vi "Temperature Check.vi"(8 "error in (no error)":errorcluster, 10 "WaitMoniter Input":T4={"Wait Time(S)"=10.0, "Chamber Temp(Deg C)"=10.0, "Chamber Temp Tolerance(%)"=10.0, "RMS Current(A)"=10.0, "RMS Current Tolerance(%)"=10.0, "Temperature Control"=FALSE, "RMS Control"=FALSE, "RMS Current Min(A)"=10.0, "RMS Current Max(A)"=10.0, "Chamber Temp Min(Deg C)"=10.0, "Chamber Temp Max(Deg C)"=10.0, "HVPPS Current Max(A)"=10.0, "HVPPS Control"=FALSE, "HVPPS Current(A)"=10.0} {"HVPPS Current(A)" format="%#_13g"; "HVPPS Current Max(A)" format="%#_13g"; "Chamber Temp Max(Deg C)" format="%#_13g"; "Chamber Temp Min(Deg C)" format="%#_13g"; "RMS Current Max(A)" format="%#_13g"; "RMS Current Min(A)" format="%#_13g"; "RMS Current Tolerance(%)" format="%#_13g"; "RMS Current(A)" format="%#_13g"; "Chamber Temp Tolerance(%)" format="%#_13g"; "Chamber Temp(Deg C)" format="%#_13g"; "Wait Time(S)" format="%#_13g"}, 11 "Data Cluster":T1={"Chamber Address"={"Starting Address"=0, "Data Length"=0}, "Modbus RTU"={"unit ID"=1, "serial type"=enum."RTU", "baud rate"=9600, "parity (even)"=2, "flow control (none)"=0, "VISA resource name"=""}, "Temparature PASS?"=FALSE, "RMS Current PASS?"=FALSE, "Ping PASS?"=FALSE, "WaitMonitor_Class"=refnum, "Status Update"="", "Test Mode"=0, "Sequence Context"=refnum, "Running?"=FALSE, "RMS_FAIL_Count"=0, "Current Temperature"=0.0, "Target Temperature"=0.0, "RMS_Current"=[], "PowerStatus"={"Chamber IP Ping"=FALSE, "RAW_Power_Status"=FALSE, "PDU1_Status_Instrument_Rack"=FALSE, "PDU2_Status_PowerSupply_Rack_1"=FALSE, "PDU3_Status_PowerSupply_Rack_2"=FALSE}, "Monitor_Interval(S)"=0.0, "Current_Monitor_Interval(S)"=0.0, "RMS_Refresh?"=FALSE, "RTD Temperature(Deg C)"=0.0, "AbortTime(S)"=0.0, "HVPPS_Current"=[], "HVPPS Current PASS?"=FALSE} {"Modbus RTU"."parity (even)" items=["None", "Odd", "Even", "Mark", "Space"]; "Modbus RTU"."flow control (none)" items=["None", "XON/XOFF", "RTS/CTS", "XON/XOFF & RTS/CTS", "DTR/DSR", "XON/XOFF & DTR/DSR"]}) -> (0 "error out":errorcluster, 3 "Data Cluster out":T1={"Chamber Address"={"Starting Address"=0, "Data Length"=0}, "Modbus RTU"={"unit ID"=1, "serial type"=enum."RTU", "baud rate"=9600, "parity (even)"=2, "flow control (none)"=0, "VISA resource name"=""}, "Temparature PASS?"=FALSE, "RMS Current PASS?"=FALSE, "Ping PASS?"=FALSE, "WaitMonitor_Class"=refnum, "Status Update"="", "Test Mode"=0, "Sequence Context"=refnum, "Running?"=FALSE, "RMS_FAIL_Count"=0, "Current Temperature"=0.0, "Target Temperature"=0.0, "RMS_Current"=[], "PowerStatus"={"Chamber IP Ping"=FALSE, "RAW_Power_Status"=FALSE, "PDU1_Status_Instrument_Rack"=FALSE, "PDU2_Status_PowerSupply_Rack_1"=FALSE, "PDU3_Status_PowerSupply_Rack_2"=FALSE}, "Monitor_Interval(S)"=0.0, "Current_Monitor_Interval(S)"=0.0, "RMS_Refresh?"=FALSE, "RTD Temperature(Deg C)"=0.0, "AbortTime(S)"=0.0, "HVPPS_Current"=[], "HVPPS Current PASS?"=FALSE} {"Modbus RTU"."parity (even)" items=["None", "Odd", "Even", "Mark", "Space"]; "Modbus RTU"."flow control (none)" items=["None", "XON/XOFF", "RTS/CTS", "XON/XOFF & RTS/CTS", "DTR/DSR", "XON/XOFF & DTR/DSR"]})   [LabVIEW 2023, in "HardwareAbstractionLayer_LVOOP.lvlib" / "Wait Monitor.lvclass"]
uses:
  Wait Monitor.lvclass
  Control/Data Cluster.ctl
  <vilib>/addons/TestStand/_TSLegacy.llb/LabVIEW Test - Sequence Context.ctl
  Teststand Steptypes/PowerMonitor/Control/PowerData.ctl
  Teststand Steptypes/WaitMoniter/Control/Moniter Step Control.ctl
  Teststand Steptypes/GlobalVariable/GlobalVariableData.vi
  Wait Monitor.lvclass/Wait Monitor.ctl
  Teststand Steptypes/LTT_TeststandSteptypes.lvlib
  <userlib>/_OpenG.lib/error/error.llb/openg_error.lvlib
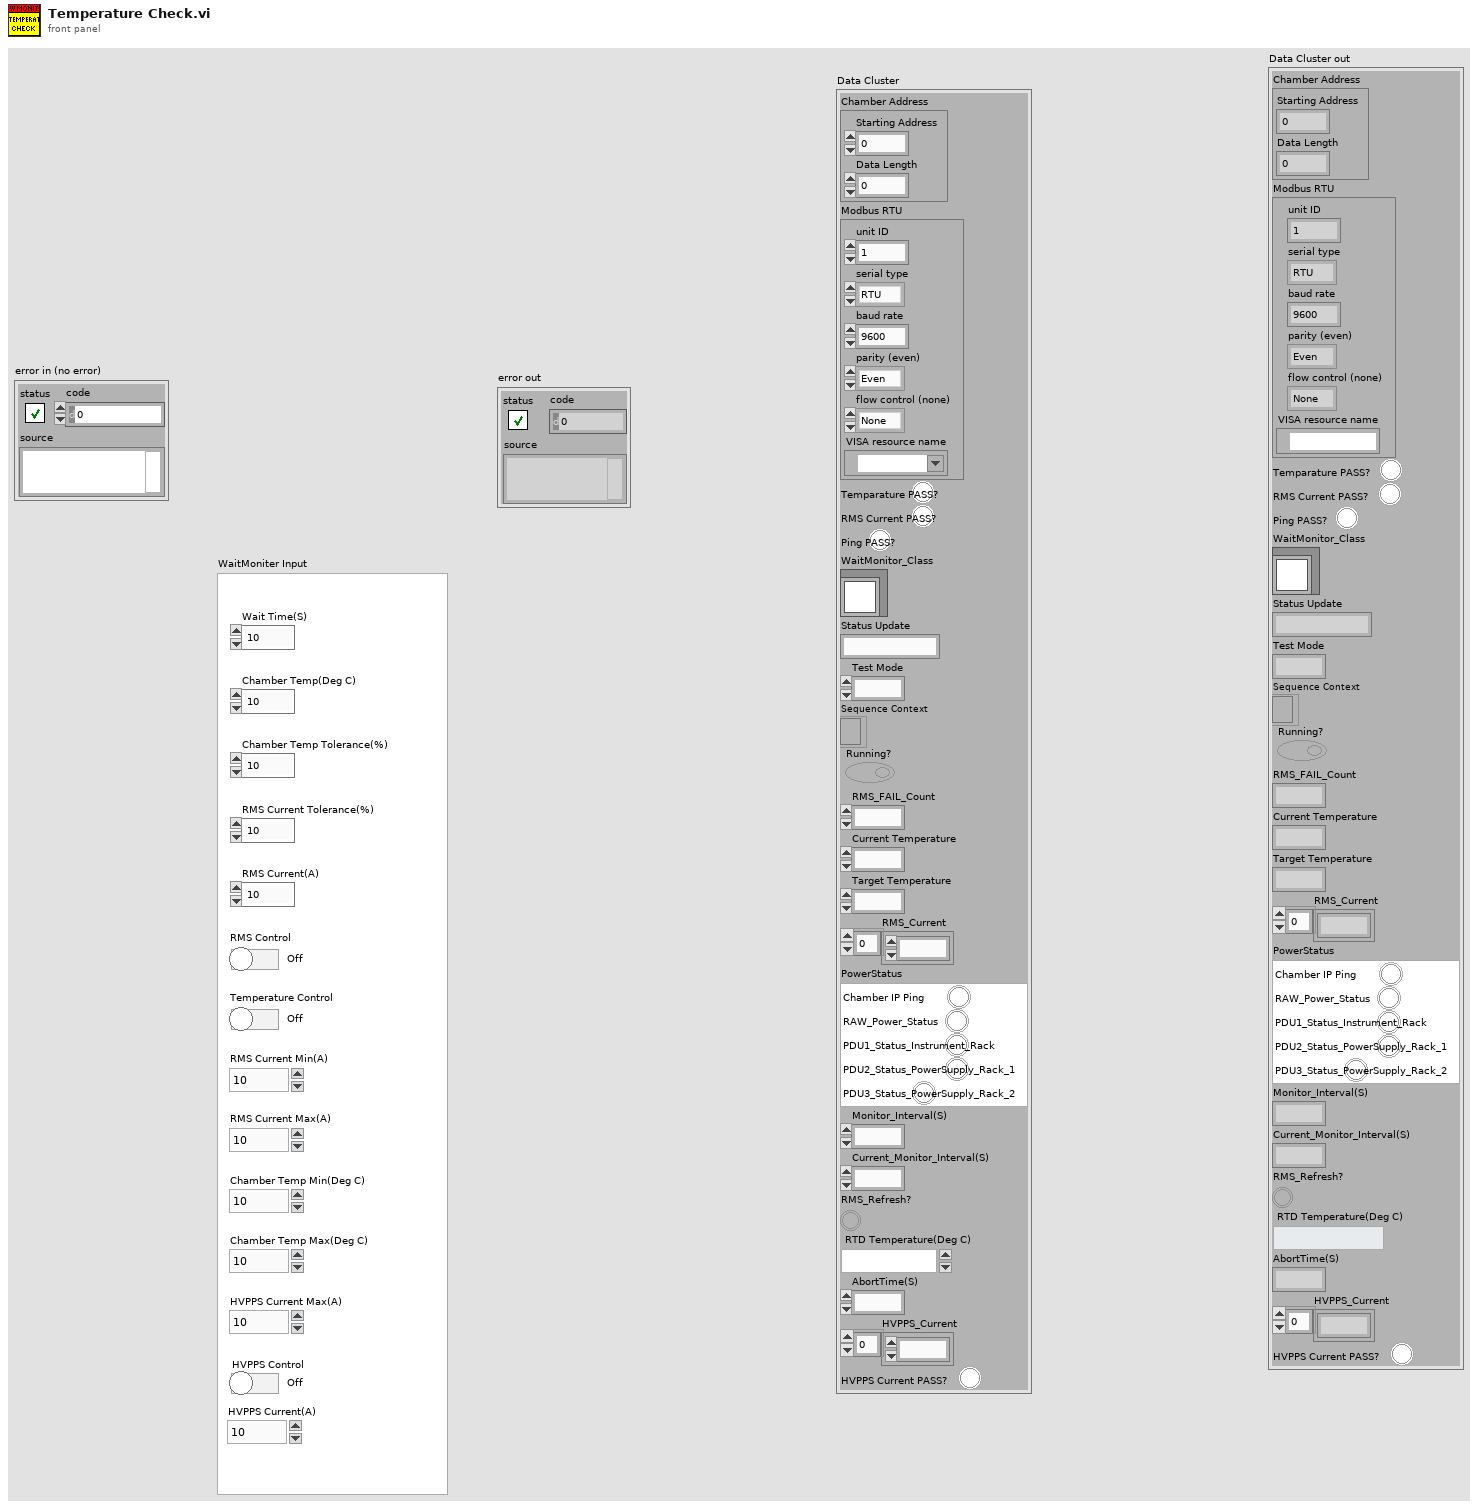
[diagram p1: front panel]
types:
  T1 = typedef "HardwareAbstractionLayer_LVOOP.lvlib/Wait Monitor.lvclass/Data Cluster.ctl" = cluster{"Chamber Address":cluster{"Starting Address":u16, "Data Length":u16}, "Modbus RTU":cluster{"unit ID":u8, "serial type":enum16{"RTU", "ASCII"}, "baud rate":u32, "parity (even)":u16, "flow control (none)":u16, "VISA resource name":refnum<visa-resource-name>}, "Temparature PASS?":bool, "RMS Current PASS?":bool, "Ping PASS?":bool, "WaitMonitor_Class":refnum<class "Wait Monitor.lvclass">, "Status Update":string, "Test Mode":u16, "Sequence Context":T2, "Running?":bool, "RMS_FAIL_Count":u16, "Current Temperature":dbl, "Target Temperature":dbl, "RMS_Current":dbl[], "PowerStatus":T3, "Monitor_Interval(S)":dbl, "Current_Monitor_Interval(S)":dbl, "RMS_Refresh?":bool, "RTD Temperature(Deg C)":dbl, "AbortTime(S)":dbl, "HVPPS_Current":dbl[], "HVPPS Current PASS?":bool}
  T2 = typedef "LabVIEW Test - Sequence Context.ctl" = refnum<k7>
  T3 = typedef "LTT_TeststandSteptypes.lvlib/PowerData.ctl" = cluster{"Chamber IP Ping":bool, "RAW_Power_Status":bool, "PDU1_Status_Instrument_Rack":bool, "PDU2_Status_PowerSupply_Rack_1":bool, "PDU3_Status_PowerSupply_Rack_2":bool}
  T4 = typedef "HardwareAbstractionLayer_LVOOP.lvlib/Wait Monitor.lvclass/Moniter Step Control.ctl" = cluster{"Wait Time(S)":dbl, "Chamber Temp(Deg C)":dbl, "Chamber Temp Tolerance(%)":dbl, "RMS Current(A)":dbl, "RMS Current Tolerance(%)":dbl, "Temperature Control":bool, "RMS Control":bool, "RMS Current Min(A)":dbl, "RMS Current Max(A)":dbl, "Chamber Temp Min(Deg C)":dbl, "Chamber Temp Max(Deg C)":dbl, "HVPPS Current Max(A)":dbl, "HVPPS Control":bool, "HVPPS Current(A)":dbl}
  T5 = cluster{"Chamber Present Temp":dbl, "Chamber Target Temp":dbl, "Chamber RTD Temp":dbl}
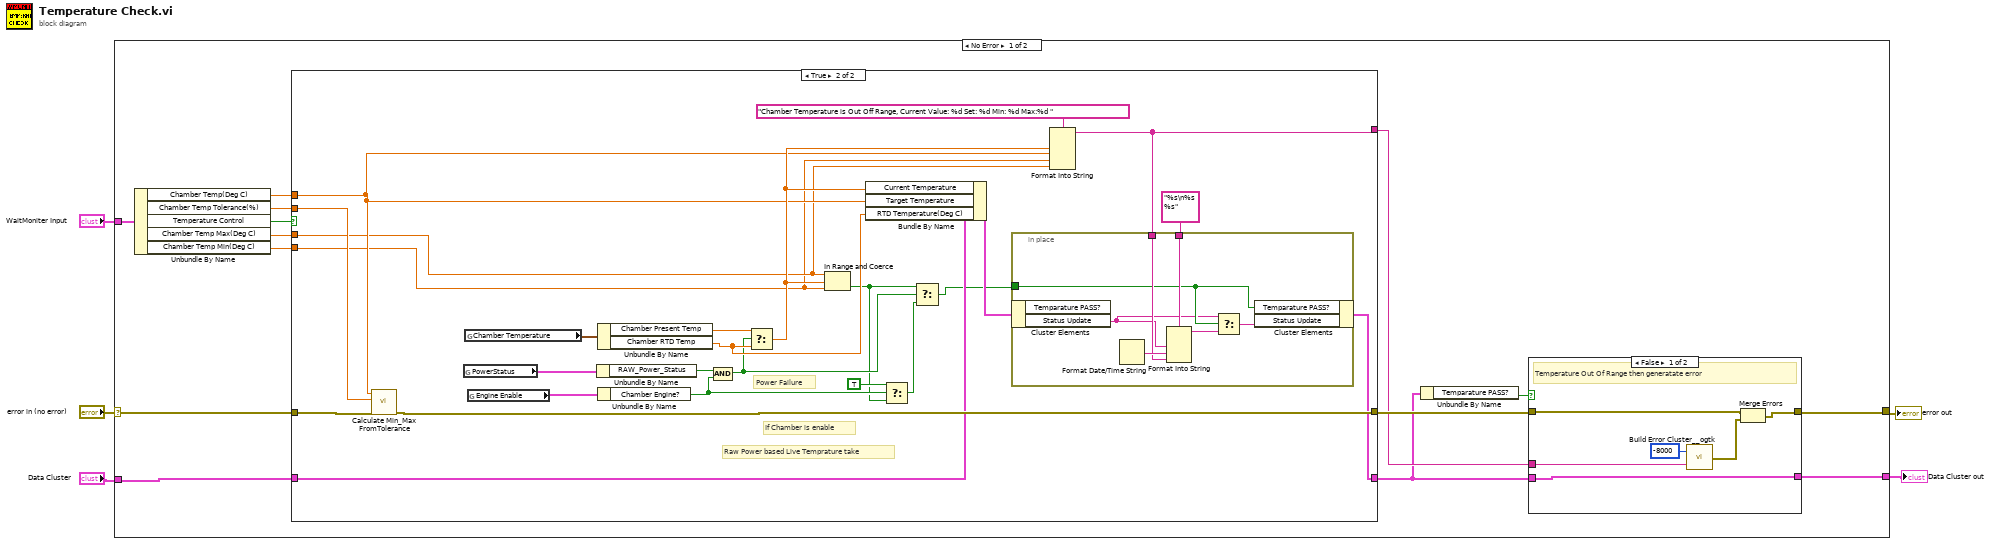
[diagram p0: block diagram]
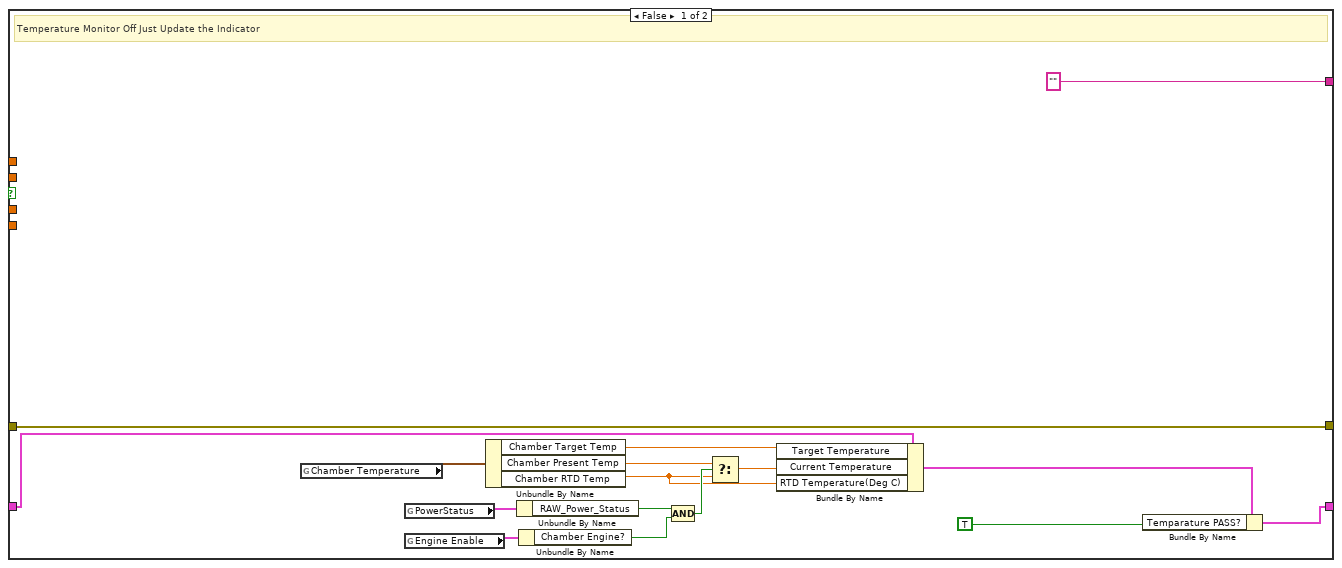
[diagram p3: hidden frame]
diagram:
  n1 = case shown="No Error" "error in (no error)" {
    selector: "error in (no error)" -> [w19 w77]
    tunnel: [w14 w77] -> w5
    tunnel: "WaitMoniter Input" -> [w13 _]
    tunnel: "Data Cluster" -> [w10 w76]
    tunnel: [w11 w76] -> w1
    frame No Error {
      n2 = Unbundle By Name(w13) -> ("Chamber Temp(Deg C)"=w18:dbl, "Chamber Temp Tolerance(%)"=w17:dbl, "Temperature Control"=w16:bool, "Chamber Temp Max(Deg C)"=w7:dbl, "Chamber Temp Min(Deg C)"=w6:dbl)
      n3 = case shown="True" w16 {
        tunnel: [w43 w66] -> w15
        tunnel: w19 -> [w43 w68]
        tunnel: w18 -> [_ w53]
        tunnel: w17 -> [_ w67]
        tunnel: ["" ("f") w57] -> w12
        tunnel: w10 -> [w31 w60]
        tunnel: [w32 w59] -> w9
        tunnel: w7 -> [_ w51]
        tunnel: w6 -> [_ w50]
        frame False {
          # "Temperature Monitor Off Just Update the Indicator"
          n4 = global read "GlobalVariableData.vi" "Chamber Temperature"() -> (w34:T5)
          n5 = global read "GlobalVariableData.vi" "PowerStatus"() -> (w35:T3)
          n6 = global read "GlobalVariableData.vi" "Engine Enable"() -> (w38:cluster{"Chamber Engine?":bool})
          n7 = Unbundle By Name(w34) -> ("Chamber Target Temp"=w29:dbl, "Chamber Present Temp"=w37:dbl, "Chamber RTD Temp"=w28:dbl)
          n8 = Unbundle By Name(w35) -> ("RAW_Power_Status"=w36:bool)
          n9 = Unbundle By Name(w38) -> ("Chamber Engine?"=w40:bool)
          n10 = Compound Arithmetic op=AND(w36, w40) -> (w39:bool)
          n11 = Select(t=w37, s=w39, f=w28) -> (s? t:f=w33:dbl)
          n12 = Bundle By Name(cluster=w31, "Target Temperature"=w29, "Current Temperature"=w33, "RTD Temperature(Deg C)"=w28) -> (w30:T1)
          n13 = Bundle By Name(cluster=w30, "Temparature PASS?"=TRUE) -> (w32:T1)
        }
        frame True {
          # "If Chamber is enable"
          # "Power Failure"
          # "Raw Power based Live Temprature take"
          n14 = call "Calculate Min_Max FromTolerance.vi"("error in"=w68, "Tolerance(%)"=w67, "Nominal Value"=w53) -> ("error out"=w66:errorcluster)  [unwired: 6 in, 2 out]
          n15 = global read "GlobalVariableData.vi" "PowerStatus"() -> (w63:T3)
          n16 = global read "GlobalVariableData.vi" "Chamber Temperature"() -> (w65:T5)
          n17 = global read "GlobalVariableData.vi" "Engine Enable"() -> (w54:cluster{"Chamber Engine?":bool})
          n18 = Unbundle By Name(w63) -> ("RAW_Power_Status"=w62:bool)
          n19 = Unbundle By Name(w65) -> ("Chamber Present Temp"=w61:dbl, "Chamber RTD Temp"=w52:dbl)
          n20 = Unbundle By Name(w54) -> ("Chamber Engine?"=w47:bool)
          n21 = Compound Arithmetic op=AND(w62, w47) -> (w49:bool)
          n22 = Select(t=w61, s=w49, f=w52) -> (s? t:f=w55:dbl)
          n23 = In Range and Coerce(upper limit=w51, x=w55, lower limit=w50) -> (In Range?=w44:bool)  [unwired: 1 out]
          n24 = Bundle By Name(cluster=w60, "Current Temperature"=w55, "Target Temperature"=w53, "RTD Temperature(Deg C)"=w52) -> (w56:T1)
          n25 = Select(t=TRUE ("f"), s=w47, f=w44) -> (s? t:f=w45:bool)
          n26 = Select(t=w44, s=w49, f=w45) -> (s? t:f=w48:bool)
          n27 = Format Into String(format string="Chamber Temperature is Out Off Range, Current Value: %d Set: %d Min: %d Max:%d ", w55, w53, w50, w51) -> (resulting string=w57:string)  [unwired: 2 in, 1 out]
          n28 = in-place {
            in-place-border: "%s\n%s %s" -> [w75]
            in-place-border: w57 -> [w73]
            in-place-border: w48 -> [w71]
            n29 = in-place-cluster #1(w56) -> ("Status Update"=w69:string)  [unwired: 1 out]
            n30 = Format Date/Time String() -> (date/time string=w74:string)  [unwired: 3 in]
            n31 = Format Into String(format string=w75, w69, w74, w73) -> (resulting string=w72:string)  [unwired: 2 in, 1 out]
            n32 = Select(t=w69, s=w71, f=w72) -> (s? t:f=w70:string)
            n33 = in-place-cluster #1("Temparature PASS?"=w71, "Status Update"=w70) -> (w59:T1)
          }
        }
      }
      n34 = Unbundle By Name(w9) -> ("Temparature PASS?"=w8:bool)
      n35 = case shown="False" w8 {
        tunnel: w15 -> [w22 w27]
        tunnel: [w20 w27] -> w14
        tunnel: w12 -> [w24 _]
        tunnel: w9 -> [w25 w26]
        tunnel: [w25 w26] -> w11
        frame False {
          # "Temperature Out Of Range then generatate error"
          n36 = call <userlib>:"Build Error Cluster__ogtk.vi"("String to Prepend to source (\"\")"=w24, "code"=-8000) -> ("error out"=w21:errorcluster)
          n37 = Merge Errors(w22, w21) -> (w20:errorcluster)
        }
        frame True {
          # "Temepearture Pass"
        }
      }
    }
    frame Error {
    }
  }
  "error out" <- w5
  "Data Cluster out" <- w1
